vi "Config Mapp.vi"(8 "error in (no error)":errorcluster, 11 "VirtualMapping":u16[][](array[numeric])) -> (0 "error out":errorcluster, 3 "VirtualMapping":u16[][](array[numeric]))   [LabVIEW 2014, in "MathLoop.lvlib"]
uses:
  MathLoop.lvlib
panel:
  in  "Stop Med":bool
  in  "Delete Med":bool
  in  "Add Med":bool
  in  "Mapping":i32(listbox)=-1 caption="Mapeo de Transductores"
  in  "Cancel Med":bool
  in  "Save Med":bool
  in  "N° Hardware:":u16
  in  "N° Transductor:":u16
  in  "Transductor Virtual:":u16
  in  "Edit Med":bool
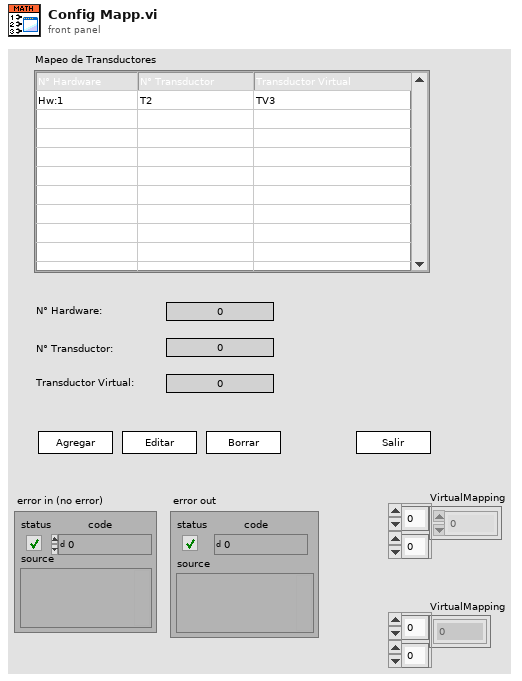
[diagram p1: front panel]
types:
  T1 = enum8{"Enabled", "Disabled", "Disabled and Grayed Out"}
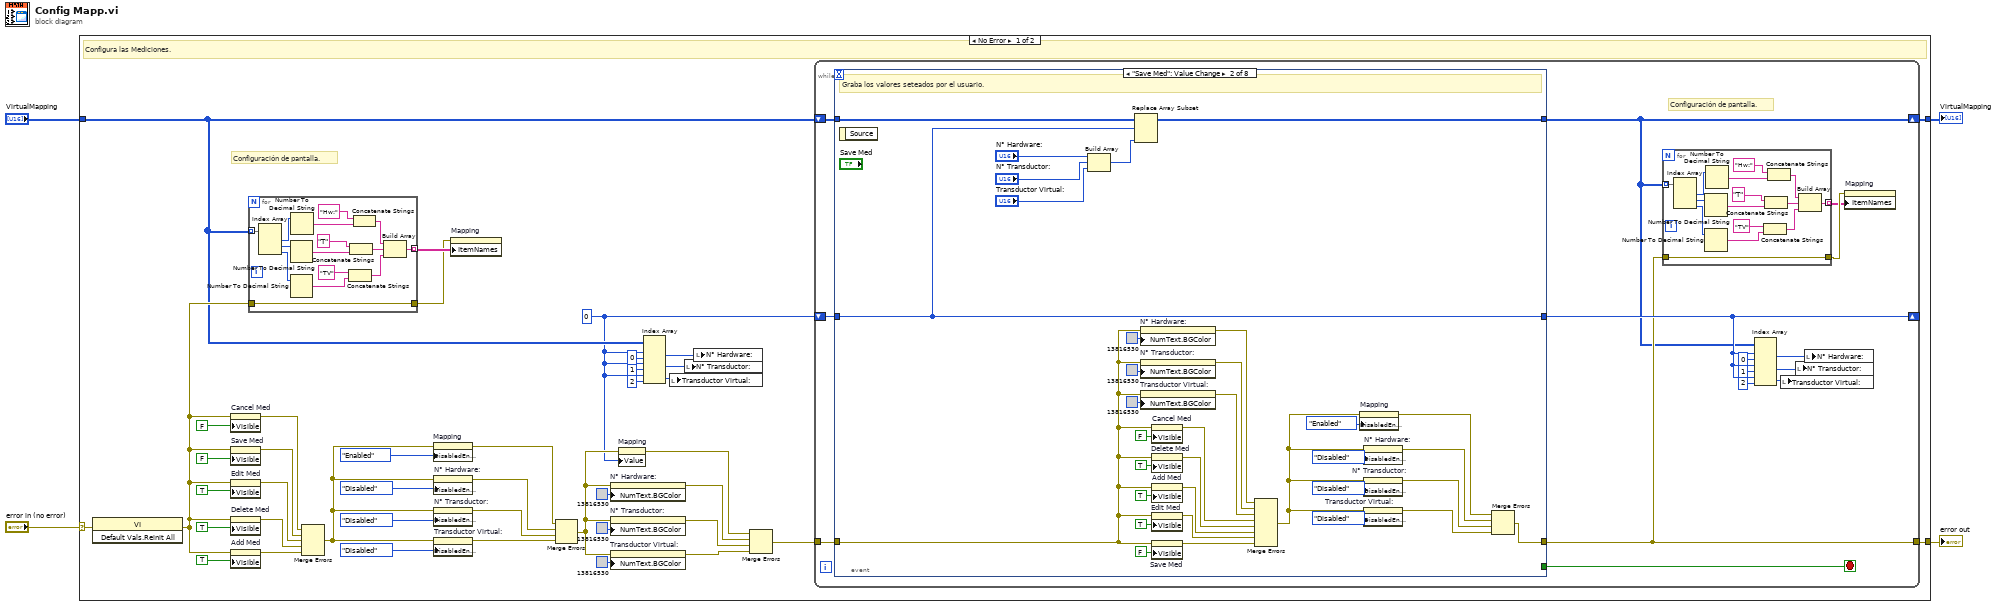
[diagram p0: block diagram]
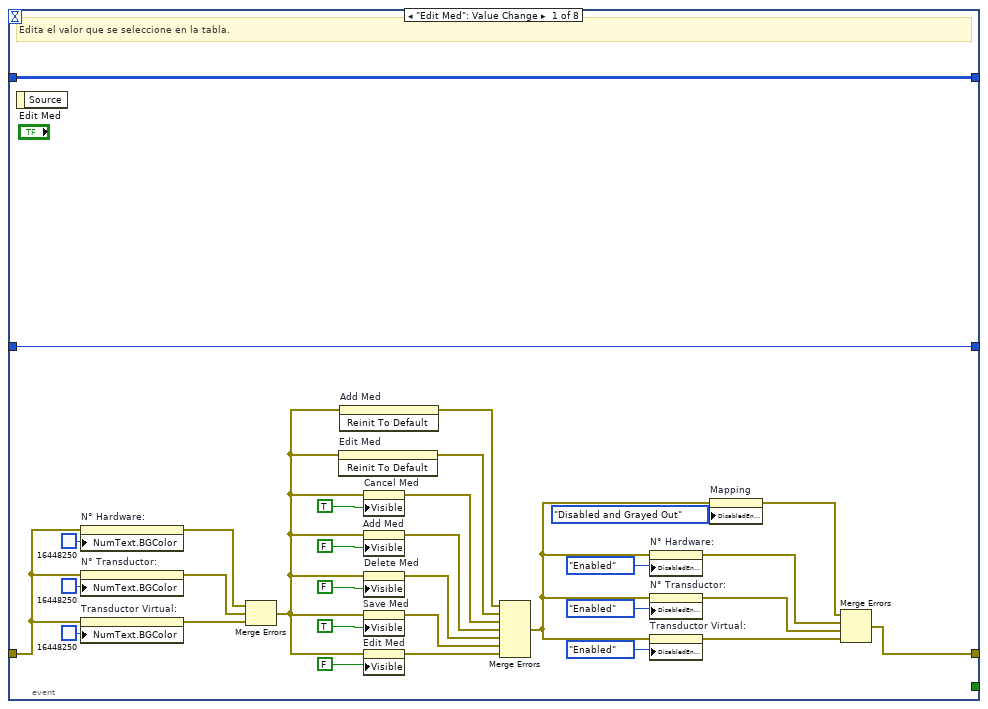
[diagram p2: hidden frame]
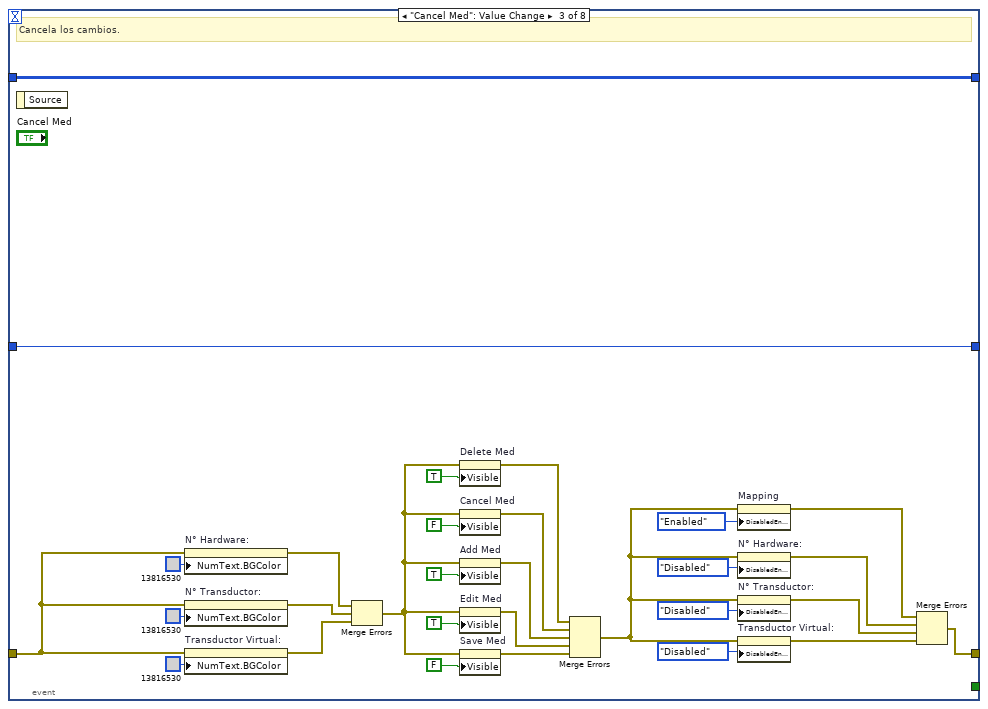
[diagram p3: hidden frame]
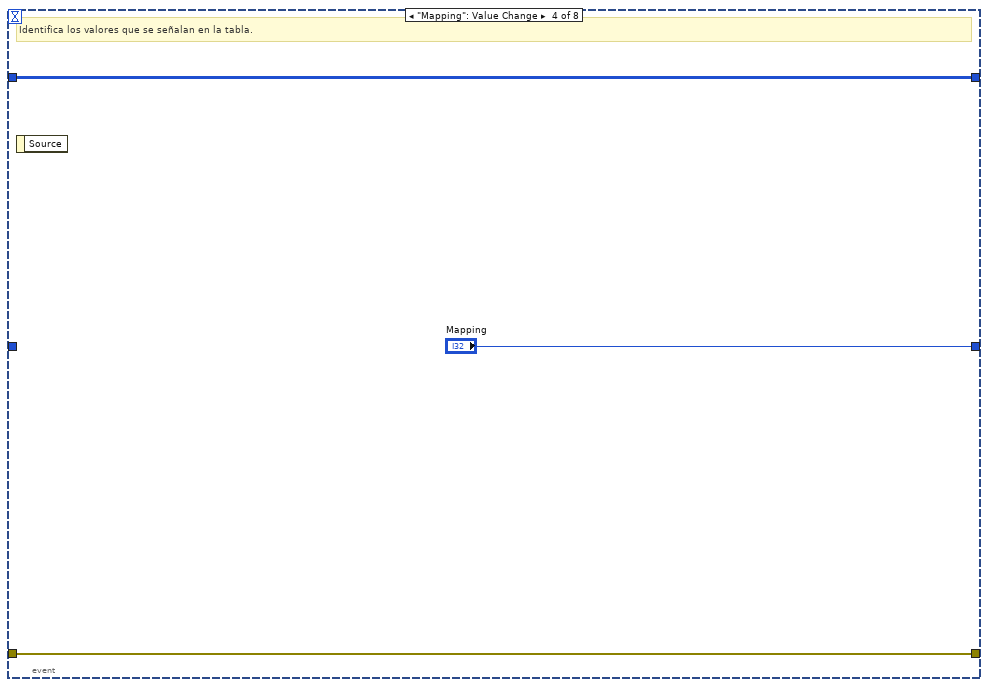
[diagram p4: hidden frame]
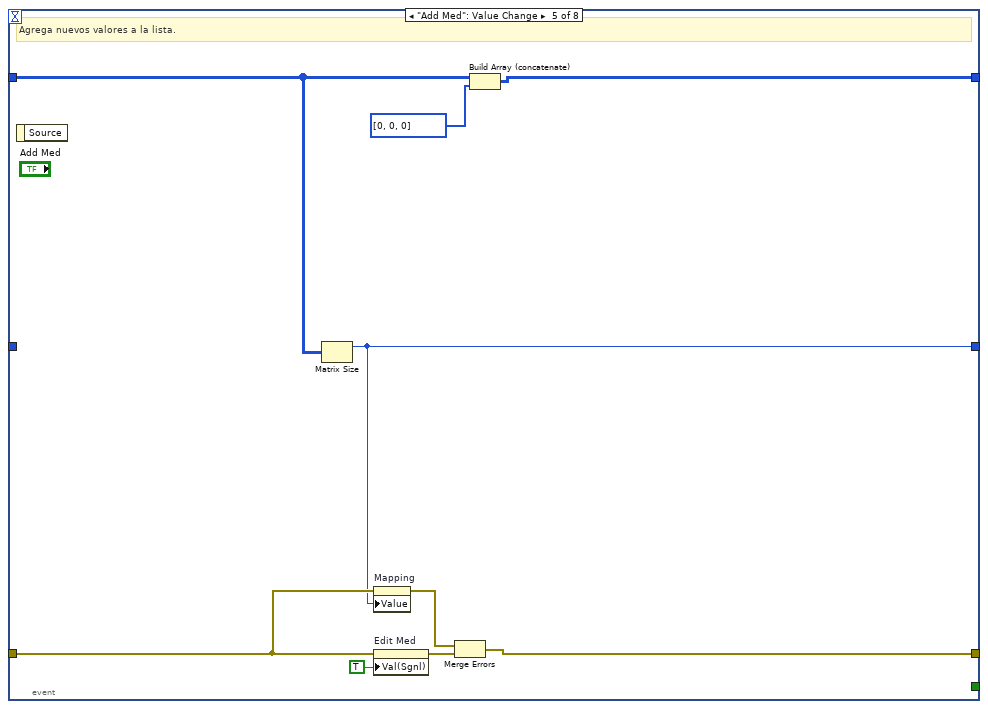
[diagram p5: hidden frame]
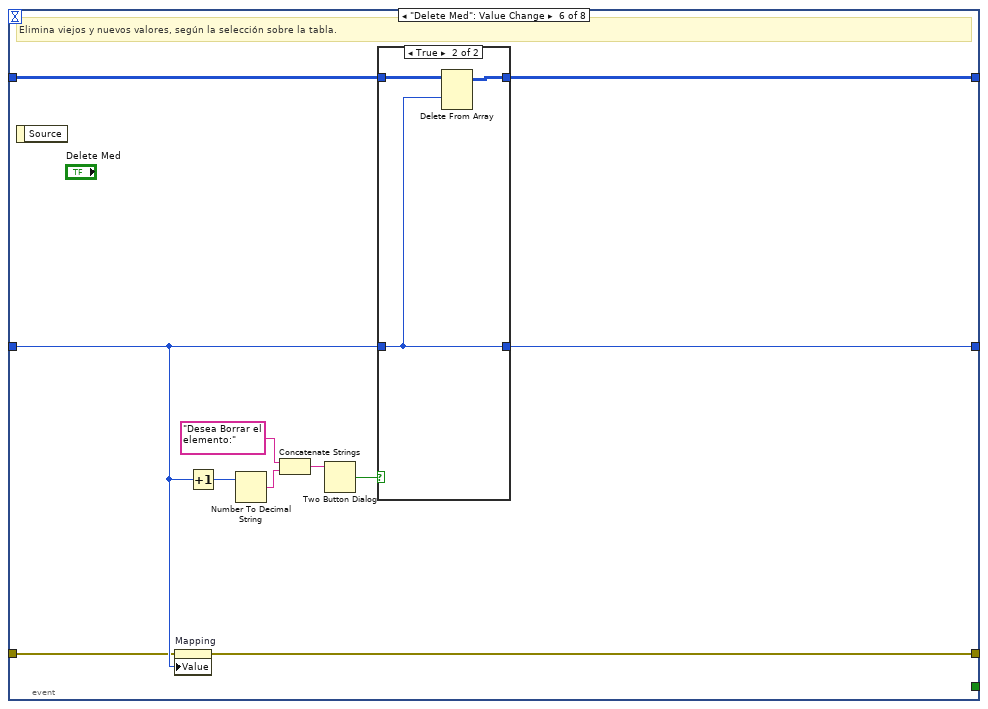
[diagram p6: hidden frame]
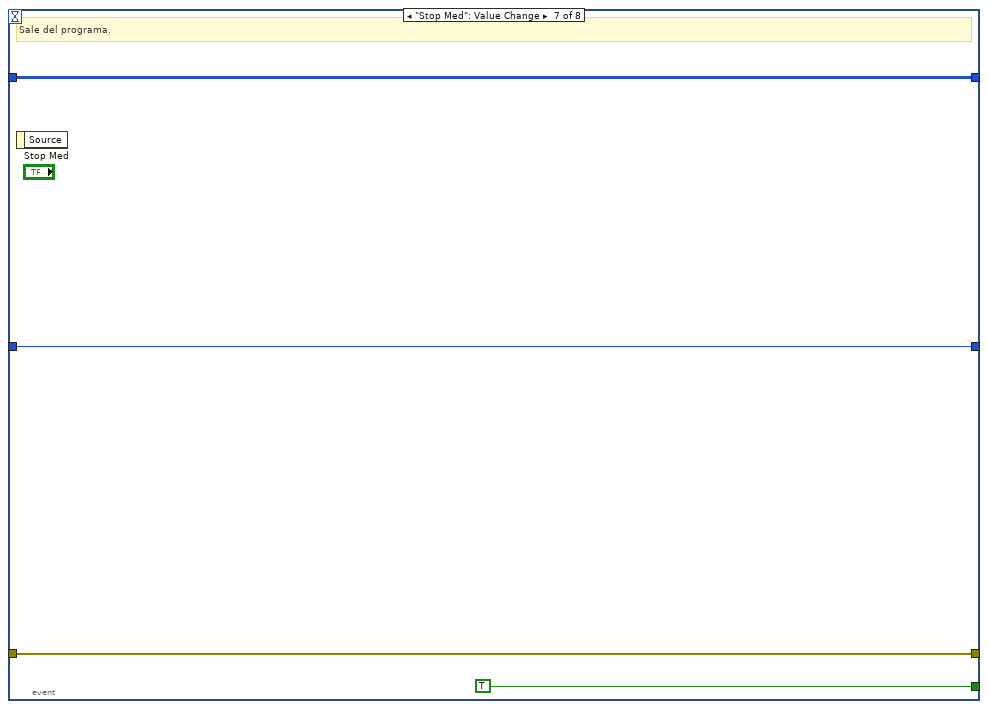
[diagram p8: hidden frame]
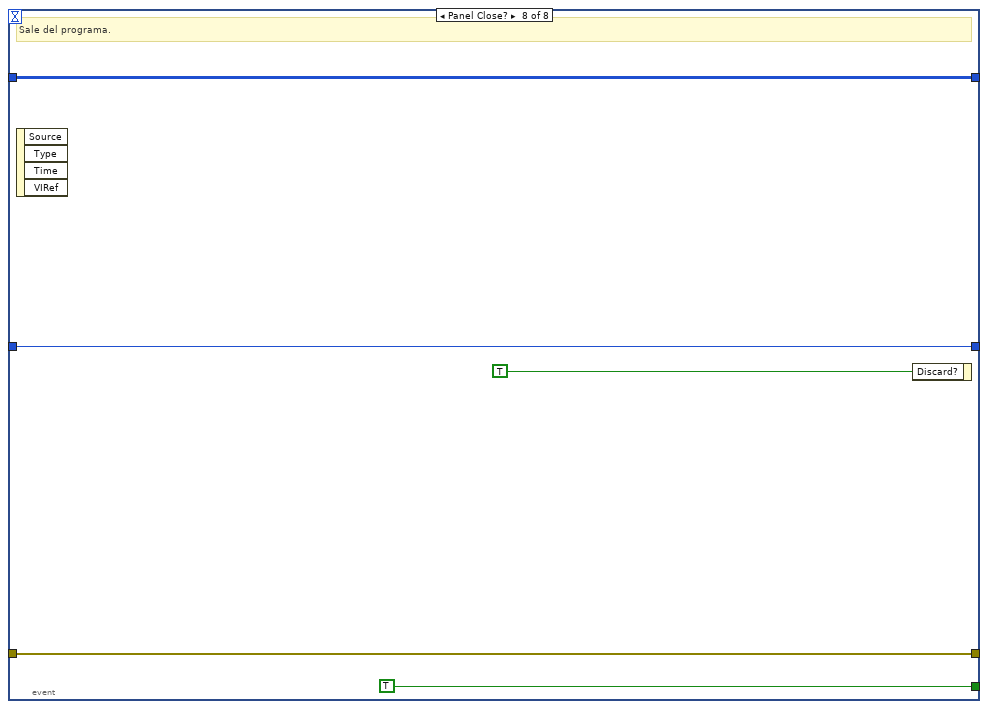
[diagram p9: hidden frame]
diagram:
  n1 = case shown="No Error" "error in (no error)" {
    selector: "error in (no error)" -> [w16 w225]
    tunnel: [w46 w225] -> w4
    tunnel: [w28 w226] -> w2
    tunnel: "VirtualMapping" -> [w6 w226]
    frame No Error {
      w5 = 0 ("disabled index (col)")
      # "Configuración de pantalla."
      # "Configura las Mediciones."
      n2 = invoke class="VI" method="Default Vals.Reinit All"(error in=w16) -> (error out=w27:errorcluster)  [unwired: 2 in, 2 out]
      n3 = property on="Cancel Med" class="Bool"(error in=w27, "Visible"=FALSE) -> (error out=w40:errorcluster)  [unwired: 1 in, 1 out]
      n4 = property on="Save Med" class="Bool"(error in=w27, "Visible"=FALSE) -> (error out=w43:errorcluster)  [unwired: 1 in, 1 out]
      n5 = property on="Edit Med" class="Bool (strict)"(error in=w27, "Visible"=TRUE) -> (error out=w42:errorcluster)  [unwired: 1 in, 1 out]
      n6 = property on="Delete Med" class="Bool"(error in=w27, "Visible"=TRUE) -> (error out=w38:errorcluster)  [unwired: 1 in, 1 out]
      n7 = property on="Add Med" class="Bool (strict)"(error in=w27, "Visible"=TRUE) -> (error out=w36:errorcluster)  [unwired: 1 in, 1 out]
      n8 = for {
        tunnel: w6 -> [w59] mode=indexing
        tunnel: w27 -> [w60]
        tunnel: [w61] -> w19 mode=indexing
        tunnel: [w60] -> w18
        n9 = Index Array(array=w59) -> (element #1=w58:u16, element #2=w57:u16, element #3=w56:u16)  [unwired: 3 in]
        n10 = Number To Decimal String(number=w57) -> (decimal integer string=w47:string)  [unwired: 1 in]
        n11 = Number To Decimal String(number=w56) -> (decimal integer string=w52:string)  [unwired: 1 in]
        n12 = Number To Decimal String(number=w58) -> (decimal integer string=w54:string)  [unwired: 1 in]
        n13 = Concatenate Strings("TV" ("element"), w52) -> (w50:string)
        n14 = Concatenate Strings("T" ("element"), w47) -> (w48:string)
        n15 = Concatenate Strings("Hw:" ("element"), w54) -> (w53:string)
        n16 = Build Array(w53, w48, w50) -> (w61:string[])
      }
      n17 = Merge Errors(w40, w43, w42, w38, w36) -> (w15:errorcluster)
      n18 = property on="Mapping" class="MCListbox (strict)"(error in=w15, "DisabledEnum"=T1."Enabled" ("Disabled")) -> (error out=w14:errorcluster)  [unwired: 1 in, 1 out]
      n19 = property on="N° Hardware:" class="DigNum (strict)"(error in=w15, "DisabledEnum"=T1."Disabled" ("Disabled")) -> (error out=w26:errorcluster)  [unwired: 1 in, 1 out]
      n20 = property on="N° Transductor:" class="DigNum (strict)"(error in=w15, "DisabledEnum"=T1."Disabled" ("Disabled")) -> (error out=w25:errorcluster)  [unwired: 1 in, 1 out]
      n21 = property on="Transductor Virtual:" class="DigNum (strict)"(error in=w15, "DisabledEnum"=T1."Disabled" ("Disabled")) -> (error out=w24:errorcluster)  [unwired: 1 in, 1 out]
      n22 = property on="Mapping" class="MCListbox (strict)"(error in=w18, "ItemNames"=w19) -> ()  [unwired: 1 in, 2 out]
      n23 = Merge Errors(w14, w26, w25, w24) -> (w20:errorcluster)
      n24 = property on="N° Hardware:" class="DigNum (strict)"(error in=w20, "NumText.BGColor"=u32 13816530) -> (error out=w30:errorcluster)  [unwired: 1 in, 1 out]
      n25 = property on="N° Transductor:" class="DigNum (strict)"(error in=w20, "NumText.BGColor"=u32 13816530) -> (error out=w31:errorcluster)  [unwired: 1 in, 1 out]
      n26 = property on="Transductor Virtual:" class="DigNum (strict)"(error in=w20, "NumText.BGColor"=u32 13816530) -> (error out=w32:errorcluster)  [unwired: 1 in, 1 out]
      n27 = property on="Mapping" class="MCListbox (strict)"(error in=w20, "Value"=w5) -> (error out=w29:errorcluster)  [unwired: 1 in, 1 out]
      n28 = Index Array(array=w6, index (row) #1=w5, index (col) #1=0 ("disabled index (col)"), index (row) #2=w5, index (col) #2=1 ("disabled index (col)"), index (row) #3=w5, index (col) #3=2 ("disabled index (col)")) -> (element #1=w9:u16, element #2=w8:u16, element #3=w7:u16)
      n29 = local write "Transductor Virtual:"(w7) -> ()
      n30 = local write "N° Transductor:"(w8) -> ()
      n31 = local write "N° Hardware:"(w9) -> ()
      n32 = Merge Errors(w29, w30, w31, w32) -> (w13:errorcluster)
      n33 = while {
        shift-right: [w62] -> w28
        shift-left: w6 -> [w74]
        shift-right: [w72] -> _
        shift-left: w5 -> [w75]
        tunnel: [w65] -> w46
        tunnel: w13 -> [w73]
        stop <- w76 stop-if-true
        # "Configuración de pantalla."
        n34 = event shown="[1] \"Save Med\": Value Change" {
          selector: _ -> [_ _ _ _ _ _ _ _]
          dyn-events: _ -> [_ _ _ _ _ _ _ _]
          timeout: _ -> [_ _ _ _ _ _ _ _]
          tunnel: w74 -> [w119 w157 w187 w190 w197 w209 w218 w224]
          tunnel: [w119 w156 w187 w190 w199 w208 w218 w224] -> w62
          tunnel: w75 -> [w92 w124 w158 _ _ w203 w216 w220]
          tunnel: w73 -> [w104 w131 w173 w189 w194 w202 w219 w222]
          tunnel: [w96 w155 w162 w189 w193 w201 w219 w222] -> w65
          tunnel: [_ _ _ _ _ _ TRUE ("Stop Med") TRUE ("Stop Med")] -> w76
          tunnel: [w92 w124 w158 "Mapping" w191 w200 w216 w220] -> w72
          event "Edit Med": Value Change {
            # "Edita el valor que se seleccione en la tabla."
            n35 = event-data() -> ()  [unwired: 1 in, 1 out]
            n36 = property on="N° Hardware:" class="DigNum (strict)"(error in=w104, "NumText.BGColor"=u32 16448250) -> (error out=w110:errorcluster)  [unwired: 1 in, 1 out]
            n37 = property on="N° Transductor:" class="DigNum (strict)"(error in=w104, "NumText.BGColor"=u32 16448250) -> (error out=w109:errorcluster)  [unwired: 1 in, 1 out]
            n38 = property on="Transductor Virtual:" class="DigNum (strict)"(error in=w104, "NumText.BGColor"=u32 16448250) -> (error out=w108:errorcluster)  [unwired: 1 in, 1 out]
            n39 = Merge Errors(w110, w109, w108) -> (w103:errorcluster)
            n40 = invoke on="Edit Med" class="Bool (strict)" method="Reinit To Default"(error in=w103) -> (error out=w112:errorcluster)  [unwired: 2 in, 2 out]
            n41 = invoke on="Add Med" class="Bool (strict)" method="Reinit To Default"(error in=w103) -> (error out=w111:errorcluster)  [unwired: 2 in, 2 out]
            n42 = property on="Cancel Med" class="Bool"(error in=w103, "Visible"=TRUE) -> (error out=w113:errorcluster)  [unwired: 1 in, 1 out]
            n43 = property on="Add Med" class="Bool (strict)"(error in=w103, "Visible"=FALSE) -> (error out=w115:errorcluster)  [unwired: 1 in, 1 out]
            n44 = property on="Delete Med" class="Bool"(error in=w103, "Visible"=FALSE) -> (error out=w117:errorcluster)  [unwired: 1 in, 1 out]
            n45 = property on="Save Med" class="Bool"(error in=w103, "Visible"=TRUE) -> (error out=w120:errorcluster)  [unwired: 1 in, 1 out]
            n46 = property on="Edit Med" class="Bool (strict)"(error in=w103, "Visible"=FALSE) -> (error out=w123:errorcluster)  [unwired: 1 in, 1 out]
            n47 = Merge Errors(w111, w112, w113, w115, w117, w120, w123) -> (w94:errorcluster)
            n48 = property on="N° Hardware:" class="DigNum (strict)"(error in=w94, "DisabledEnum"=T1."Enabled" ("Disabled")) -> (error out=w97:errorcluster)  [unwired: 1 in, 1 out]
            n49 = property on="N° Transductor:" class="DigNum (strict)"(error in=w94, "DisabledEnum"=T1."Enabled" ("Disabled")) -> (error out=w98:errorcluster)  [unwired: 1 in, 1 out]
            n50 = property on="Transductor Virtual:" class="DigNum (strict)"(error in=w94, "DisabledEnum"=T1."Enabled" ("Disabled")) -> (error out=w99:errorcluster)  [unwired: 1 in, 1 out]
            n51 = property on="Mapping" class="MCListbox (strict)"(error in=w94, "DisabledEnum"=T1."Disabled and Grayed Out" ("Disabled")) -> (error out=w93:errorcluster)  [unwired: 1 in, 1 out]
            n52 = Merge Errors(w93, w97, w98, w99) -> (w96:errorcluster)
          }
          event "Save Med": Value Change {
            # "Graba los valores seteados por el usuario."
            n53 = event-data() -> ()  [unwired: 1 in, 1 out]
            n54 = Build Array("N° Hardware:", "N° Transductor:", "Transductor Virtual:") -> (w132:u16[])
            n55 = Replace Array Subset(array=w157, new element=w132, index (row)=w124) -> (w156:u16[][])  [unwired: 1 in]
            n56 = property on="N° Hardware:" class="DigNum (strict)"(error in=w131, "NumText.BGColor"=u32 13816530) -> (error out=w127:errorcluster)  [unwired: 1 in, 1 out]
            n57 = property on="N° Transductor:" class="DigNum (strict)"(error in=w131, "NumText.BGColor"=u32 13816530) -> (error out=w128:errorcluster)  [unwired: 1 in, 1 out]
            n58 = property on="Transductor Virtual:" class="DigNum (strict)"(error in=w131, "NumText.BGColor"=u32 13816530) -> (error out=w129:errorcluster)  [unwired: 1 in, 1 out]
            n59 = property on="Cancel Med" class="Bool"(error in=w131, "Visible"=FALSE) -> (error out=w153:errorcluster)  [unwired: 1 in, 1 out]
            n60 = property on="Delete Med" class="Bool"(error in=w131, "Visible"=TRUE) -> (error out=w154:errorcluster)  [unwired: 1 in, 1 out]
            n61 = property on="Add Med" class="Bool (strict)"(error in=w131, "Visible"=TRUE) -> (error out=w150:errorcluster)  [unwired: 1 in, 1 out]
            n62 = property on="Edit Med" class="Bool (strict)"(error in=w131, "Visible"=TRUE) -> (error out=w145:errorcluster)  [unwired: 1 in, 1 out]
            n63 = property on="Save Med" class="Bool"(error in=w131, "Visible"=FALSE) -> (error out=w146:errorcluster)  [unwired: 1 in, 1 out]
            n64 = Merge Errors(w127, w128, w129, w153, w154, w150, w145, w146) -> (w134:errorcluster)
            n65 = property on="Mapping" class="MCListbox (strict)"(error in=w134, "DisabledEnum"=T1."Enabled" ("Disabled")) -> (error out=w130:errorcluster)  [unwired: 1 in, 1 out]
            n66 = property on="N° Hardware:" class="DigNum (strict)"(error in=w134, "DisabledEnum"=T1."Disabled" ("Disabled")) -> (error out=w136:errorcluster)  [unwired: 1 in, 1 out]
            n67 = property on="N° Transductor:" class="DigNum (strict)"(error in=w134, "DisabledEnum"=T1."Disabled" ("Disabled")) -> (error out=w137:errorcluster)  [unwired: 1 in, 1 out]
            n68 = property on="Transductor Virtual:" class="DigNum (strict)"(error in=w134, "DisabledEnum"=T1."Disabled" ("Disabled")) -> (error out=w138:errorcluster)  [unwired: 1 in, 1 out]
            n69 = Merge Errors(w130, w136, w137, w138) -> (w155:errorcluster)
          }
          event "Cancel Med": Value Change {
            # "Cancela los cambios."
            n70 = event-data() -> ()  [unwired: 1 in, 1 out]
            n71 = property on="N° Hardware:" class="DigNum (strict)"(error in=w173, "NumText.BGColor"=u32 13816530) -> (error out=w169:errorcluster)  [unwired: 1 in, 1 out]
            n72 = property on="N° Transductor:" class="DigNum (strict)"(error in=w173, "NumText.BGColor"=u32 13816530) -> (error out=w170:errorcluster)  [unwired: 1 in, 1 out]
            n73 = property on="Transductor Virtual:" class="DigNum (strict)"(error in=w173, "NumText.BGColor"=u32 13816530) -> (error out=w171:errorcluster)  [unwired: 1 in, 1 out]
            n74 = Merge Errors(w169, w170, w171) -> (w172:errorcluster)
            n75 = property on="Delete Med" class="Bool"(error in=w172, "Visible"=TRUE) -> (error out=w178:errorcluster)  [unwired: 1 in, 1 out]
            n76 = property on="Cancel Med" class="Bool"(error in=w172, "Visible"=FALSE) -> (error out=w177:errorcluster)  [unwired: 1 in, 1 out]
            n77 = property on="Add Med" class="Bool (strict)"(error in=w172, "Visible"=TRUE) -> (error out=w181:errorcluster)  [unwired: 1 in, 1 out]
            n78 = property on="Edit Med" class="Bool (strict)"(error in=w172, "Visible"=TRUE) -> (error out=w186:errorcluster)  [unwired: 1 in, 1 out]
            n79 = property on="Save Med" class="Bool"(error in=w172, "Visible"=FALSE) -> (error out=w185:errorcluster)  [unwired: 1 in, 1 out]
            n80 = Merge Errors(w178, w177, w181, w186, w185) -> (w160:errorcluster)
            n81 = property on="Mapping" class="MCListbox (strict)"(error in=w160, "DisabledEnum"=T1."Enabled" ("Disabled")) -> (error out=w159:errorcluster)  [unwired: 1 in, 1 out]
            n82 = property on="N° Hardware:" class="DigNum (strict)"(error in=w160, "DisabledEnum"=T1."Disabled" ("Disabled")) -> (error out=w163:errorcluster)  [unwired: 1 in, 1 out]
            n83 = property on="N° Transductor:" class="DigNum (strict)"(error in=w160, "DisabledEnum"=T1."Disabled" ("Disabled")) -> (error out=w164:errorcluster)  [unwired: 1 in, 1 out]
            n84 = property on="Transductor Virtual:" class="DigNum (strict)"(error in=w160, "DisabledEnum"=T1."Disabled" ("Disabled")) -> (error out=w165:errorcluster)  [unwired: 1 in, 1 out]
            n85 = Merge Errors(w159, w163, w164, w165) -> (w162:errorcluster)
          }
          event "Mapping": Value Change {
            # "Identifica los valores que se señalan en la tabla."
            n86 = event-data() -> ()  [unwired: 1 in, 1 out]
          }
          event "Add Med": Value Change {
            # "Agrega nuevos valores a la lista."
            n87 = event-data() -> ()  [unwired: 1 in, 1 out]
            n88 = Matrix Size(0:w197) -> (1:w191:i32)  [unwired: 1 out]
            n89 = property on="Mapping" class="MCListbox (strict)"(error in=w194, "Value"=w191) -> (error out=w196:errorcluster)  [unwired: 1 in, 1 out]
            n90 = property on="Edit Med" class="Bool (strict)"(error in=w194, "Val(Sgnl)"=TRUE) -> (error out=w195:errorcluster)  [unwired: 1 in, 1 out]
            n91 = Merge Errors(w196, w195) -> (w193:errorcluster)
            n92 = Build Array (concatenate)(w197, u16[] [0, 0, 0] ("element")) -> (w199:u16[][])
          }
          event "Delete Med": Value Change {
            # "Elimina viejos y nuevos valores, según la selección sobre la tabla."
            n93 = event-data() -> ()  [unwired: 1 in, 1 out]
            n94 = property on="Mapping" class="MCListbox (strict)"(error in=w202, "Value"=w203) -> (error out=w201:errorcluster)  [unwired: 1 in, 1 out]
            n95 = Increment(x=w203) -> (x+1=w204:i32)
            n96 = Number To Decimal String(number=w204) -> (decimal integer string=w206:string)  [unwired: 1 in]
            n97 = Concatenate Strings("Desea Borrar el elemento:" ("message"), w206) -> (w205:string)
            n98 = Two Button Dialog(message=w205) -> (T button?=w210:bool)  [unwired: 2 in]
            n99 = case shown="True" w210 {
              tunnel: w209 -> [w211 w215]
              tunnel: [w212 w213] -> w200
              tunnel: w203 -> [w212 w213]
              tunnel: [w211 w214] -> w208
              frame False {
              }
              frame True {
                n100 = Delete From Array(array=w215, index (row)=w213) -> (array with subset deleted=w214:u16[][])  [unwired: 2 in, 1 out]
              }
            }
          }
          event "Stop Med": Value Change {
            # "Sale del programa."
            n101 = event-data() -> ()  [unwired: 1 in, 1 out]
          }
          event Panel Close? {
            # "Sale del programa."
            n102 = event-data() -> ()  [unwired: 1 in, 4 out]
            n103 = event-data("Discard?"=TRUE) -> ()  [unwired: 1 in, 1 out]
          }
        }
        n104 = for {
          tunnel: w62 -> [w89] mode=indexing
          tunnel: w65 -> [w90]
          tunnel: [w91] -> w63 mode=indexing
          tunnel: [w90] -> w64
          n105 = Index Array(array=w89) -> (element #1=w88:u16, element #2=w87:u16, element #3=w86:u16)  [unwired: 3 in]
          n106 = Number To Decimal String(number=w87) -> (decimal integer string=w77:string)  [unwired: 1 in]
          n107 = Number To Decimal String(number=w86) -> (decimal integer string=w82:string)  [unwired: 1 in]
          n108 = Number To Decimal String(number=w88) -> (decimal integer string=w84:string)  [unwired: 1 in]
          n109 = Concatenate Strings("TV" ("element"), w82) -> (w80:string)
          n110 = Concatenate Strings("T" ("element"), w77) -> (w78:string)
          n111 = Concatenate Strings("Hw:" ("element"), w84) -> (w83:string)
          n112 = Build Array(w83, w78, w80) -> (w91:string[])
        }
        n113 = Index Array(array=w62, index (row) #1=w72, index (col) #1=0 ("disabled index (col)"), index (row) #2=w72, index (col) #2=1 ("disabled index (col)"), index (row) #3=w72, index (col) #3=2 ("disabled index (col)")) -> (element #1=w68:u16, element #2=w67:u16, element #3=w66:u16)
        n114 = local write "Transductor Virtual:"(w66) -> ()
        n115 = local write "N° Transductor:"(w67) -> ()
        n116 = local write "N° Hardware:"(w68) -> ()
        n117 = property on="Mapping" class="MCListbox (strict)"(error in=w64, "ItemNames"=w63) -> ()  [unwired: 1 in, 2 out]
      }
    }
    frame Error {
    }
  }
  "VirtualMapping" <- w2
  "error out" <- w4
